vi "Valve2BoardChannel.vi"(11 "ValveID":u16(ring) items=["A1", "A2", "A3", "A4", "B1", "B2", "B3", "B4", "B5", "B6", "B7", "B8", "A5", "A6", "A7", "A8"]) -> (2 "Channel":enum16{"1", "2", "3", "4", "5", "6", "7", "8"}(ring), 3 "Flowboard":enum16{"A", "B", "C"}(ring))   [LabVIEW 2016]
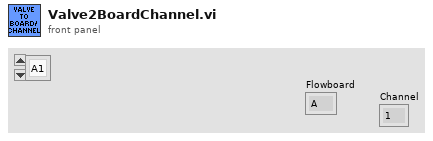
[diagram p1: front panel]
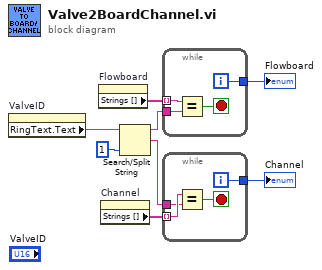
[diagram p0: block diagram]
diagram:
  n1 = property on="ValveID" class="Ring (strict)"() -> ("RingText.Text"=w8:string)  [unwired: 2 in, 2 out]
  n2 = property on="Flowboard" class="Enum (strict)"() -> ("Strings []"=w6:string[])  [unwired: 2 in, 2 out]
  n3 = property on="Channel" class="Enum (strict)"() -> ("Strings []"=w4:string[])  [unwired: 2 in, 2 out]
  n4 = Search/Split String(string=w8, offset (0)=1) -> (substring before match=w5:string, match + rest of string=w3:string)  [unwired: 1 in, 1 out]
  n5 = while {
    tunnel: w6 -> [w12] mode=indexing
    tunnel: w5 -> [w11]
    tunnel: [w9] -> w1
    i -> [w9]
    stop <- w10 stop-if-true
    n6 = Equal?(x=w12, y=w11) -> (x = y?=w10:bool)
  }
  "Flowboard" <- w1
  n7 = while {
    tunnel: w4 -> [w16] mode=indexing
    tunnel: w3 -> [w15]
    tunnel: [w13] -> w2
    i -> [w13]
    stop <- w14 stop-if-true
    n8 = Equal?(x=w16, y=w15) -> (x = y?=w14:bool)
  }
  "Channel" <- w2
